vi "Host - Set Slave State.vi"(7 "timeout":u32, 8 "error in (no error)":errorcluster, 9 "ackError":bool=TRUE, 10 "slaveState":u32(ring)=1 items=["Init"=1, "PreOP"=2, "BootStrap"=3, "SafeOP"=4, "OP"=8], 11 "Slave Ref in":refnum<k21>) -> (0 "error out":errorcluster, 1 "statusCode":u16, 2 "appSpecCode":u8, 3 "Slave Ref out":refnum<k21>)   [LabVIEW 2016, in "Scan Engine Custom Device.lvlib"]
uses:
  Scan Engine Custom Device.lvlib
  <resource>/objmgr/IndComECAT.rc
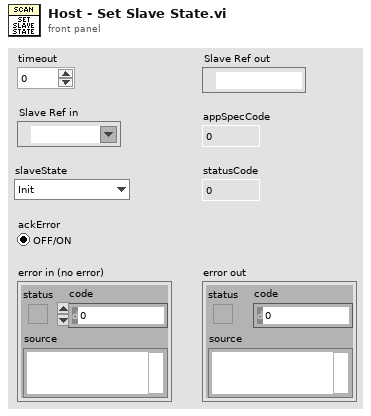
[diagram p1: front panel]
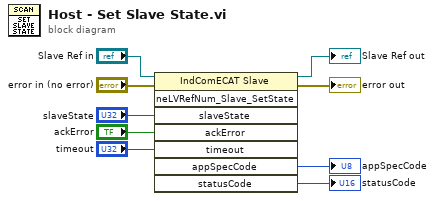
[diagram p0: block diagram]
diagram:
  n1 = invoke class="IndComECAT Slave" method="neLVRefNum_Slave_SetState"(reference="Slave Ref in", error in="error in (no error)", "slaveState"="slaveState", "ackError"="ackError", "timeout"="timeout") -> (reference out=→"Slave Ref out":refnum<k21>, error out=→"error out":errorcluster, "appSpecCode"=→"appSpecCode":u8, "statusCode"=→"statusCode":u16)  [unwired: 3 in, 4 out]
